vi "Encoder Voltage to Angle.vi"(11 "Encoder Voltages":dbl[](array[numeric])) -> (3 "Angle":dbl[](array[numeric]))   [LabVIEW 2020]
doc: "Converts the absolute encoder analog input voltages to degrees [0,360]."
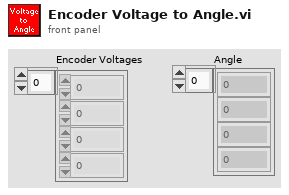
[diagram p1: front panel]
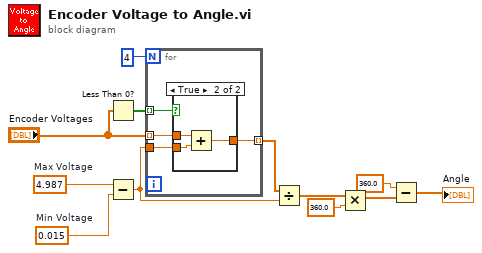
[diagram p0: block diagram]
diagram:
  w5 = 0.015  # Min Voltage
  w6 = 4.987  # Max Voltage
  n1 = Less Than 0?(x="Encoder Voltages") -> (x < 0?=w9:bool[])
  n2 = Subtract(x=w6, y=w5) -> (x-y=w7:dbl)
  n3 = for {
    N: 4 -> [_]
    tunnel: w9 -> [w13] mode=indexing
    tunnel: "Encoder Voltages" -> [w16] mode=indexing
    tunnel: w7 -> [w15]
    tunnel: [w14] -> w8 mode=indexing
    n4 = case shown="True" w13 {
      tunnel: w16 -> [w17 w19]
      tunnel: w15 -> [_ w20]
      tunnel: [w17 w18] -> w14
      frame False {
      }
      frame True {
        n5 = Add(x=w19, y=w20) -> (x+y=w18:dbl)
      }
    }
  }
  n6 = Divide(x=w8, y=w7) -> (x/y=w12:dbl[])
  n7 = Multiply(x=w12, y=360.0) -> (x*y=w2:dbl[])
  n8 = Subtract(x=360.0 ("y"), y=w2) -> (x-y=→"Angle":dbl[])
